vi "_script_fix_Parse State Queue in Find Parse State Queue vi name.vi"   [LabVIEW 2014]
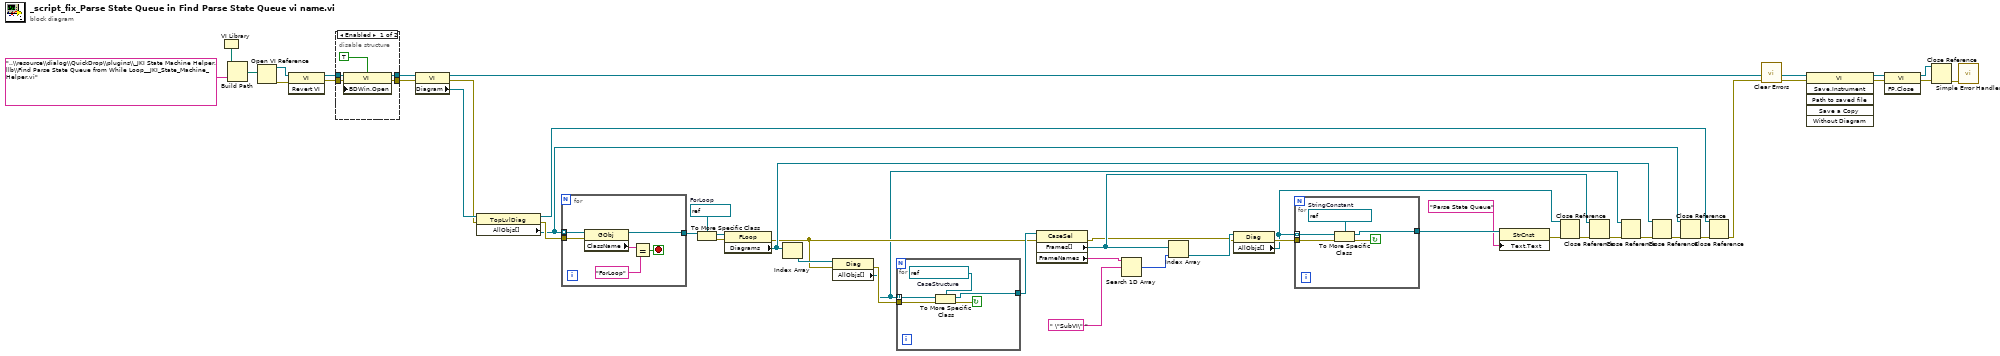
[diagram p0: block diagram]
diagram:
  w37 = refnum<vi> refnum  # ForLoop
  n1 = VI Library() -> (path=w46:path)
  n2 = Build Path(base path=w46, name or relative path="..\\resource\\dialog\\QuickDrop\\plugins\\_JKI State Machine Helper.llb\\Find Parse State Queue from While Loop__JKI_State_Machine_Helper.vi") -> (appended path=w44:path)
  n3 = Open VI Reference(vi path=w44) -> (vi reference=w47:refnum<vi>, error out=w48:errorcluster)  [unwired: 5 in]
  n4 = invoke class="VI" method="Revert VI"(reference=w47, error in=w48) -> (reference out=w24:refnum<vi>, error out=w23:errorcluster)  [unwired: 1 in, 1 out]
  n5 = disable-structure shown="Enabled" {
    disable-tunnel: w24 -> [w53 w55]
    disable-tunnel: w23 -> [w52 w54]
    disable-tunnel: [w51 w55] -> w22
    disable-tunnel: [w50 w54] -> w21
    frame Enabled {
      n6 = property class="VI"(reference=w53, error in=w52, "BDWin.Open"=TRUE ("Block Diagram Window:Open")) -> (reference out=w51:refnum<vi>, error out=w50:errorcluster)
    }
    frame Disabled {
    }
  }
  n7 = property class="VI"(reference=w22, error in=w21) -> (reference out=w43:refnum<vi>, error out=w40:errorcluster, "Diagram"=w41:refnum<vi>)
  n8 = property class="TopLvlDiag"(reference=w41, error in=w40) -> (reference out=w26:refnum<vi>, error out=w39:errorcluster, "AllObjs[]"=w28:refnum<vi>[])
  n9 = for {
    tunnel: w28 -> [w61] mode=indexing
    tunnel: w39 -> [w60]
    tunnel: [w59] -> w38
    stop <- w56 stop-if-true
    n10 = property class="GObj"(reference=w61, error in=w60) -> (reference out=w59:refnum<vi>, "ClassName"=w58:string)  [unwired: 1 out]
    n11 = Equal?(x=w58, y="ForLoop") -> (x = y?=w56:bool)
  }
  n12 = To More Specific Class(target class=w37, reference=w38) -> (specific class reference=w36:refnum<vi>, error out=w35:errorcluster)  [unwired: 1 in]
  n13 = property class="FLoop"(reference=w36, error in=w35) -> (error out=w16:errorcluster, "Diagrams"=w20:refnum<vi>[])  [unwired: 1 out]
  n14 = Index Array(array=w20) -> (element=w19:refnum<vi>)  [unwired: 1 in]
  n15 = property class="Diag"(reference=w19, error in=w16) -> (error out=w18:errorcluster, "AllObjs[]"=w12:refnum<vi>[])  [unwired: 1 out]
  n16 = for {
    tunnel: w12 -> [w66] mode=indexing
    tunnel: w18 -> [w65]
    tunnel: [w63] -> w17
    stop <- w64 continue-if-true
    w62 = refnum<vi> refnum  # CaseStructure
    n17 = To More Specific Class(target class=w62, reference=w66, error in=w65) -> (specific class reference=w63:refnum<vi>, error out=w64:errorcluster)
  }
  n18 = property class="CaseSel"(reference=w17, error in=w16) -> (error out=w6:errorcluster, "Frames[]"=w9:refnum<vi>[], "FrameNames"=w11:string[])  [unwired: 1 out]
  n19 = Search 1D Array(1D array=w11, element=" \"SubVI\" " ("y")) -> (index of element=w8:i32)  [unwired: 1 in]
  n20 = Index Array(array=w9, index=w8) -> (element=w7:refnum<vi>)
  n21 = property class="Diag"(reference=w7, error in=w6) -> (error out=w34:errorcluster, "AllObjs[]"=w30:refnum<vi>[])  [unwired: 1 out]
  n22 = for {
    tunnel: w30 -> [w71] mode=indexing
    tunnel: w34 -> [w70]
    tunnel: [w67] -> w33
    stop <- w68 continue-if-true
    w69 = refnum<vi> refnum  # StringConstant
    n23 = To More Specific Class(target class=w69, reference=w71, error in=w70) -> (specific class reference=w67:refnum<vi>, error out=w68:errorcluster)
  }
  n24 = property class="StrCnst"(reference=w33, "Text.Text"="Parse State Queue") -> (error out=w31:errorcluster)  [unwired: 1 in, 1 out]
  n25 = Close Reference(reference=w30, error in (no error)=w31) -> (error out=w15:errorcluster)
  n26 = Close Reference(reference=w9, error in (no error)=w15) -> (error out=w14:errorcluster)
  n27 = Close Reference(reference=w12, error in (no error)=w14) -> (error out=w13:errorcluster)
  n28 = Close Reference(reference=w20, error in (no error)=w13) -> (error out=w29:errorcluster)
  n29 = Close Reference(reference=w28, error in (no error)=w29) -> (error out=w27:errorcluster)
  n30 = Close Reference(reference=w26, error in (no error)=w27) -> (error out=w25:errorcluster)
  n31 = call <vilib>:"Clear Errors.vi"("error in (no error)"=w25) -> ("error out"=w1:errorcluster)  [unwired: 6 in]
  n32 = invoke class="VI" method="Save.Instrument"(reference=w43, error in=w1) -> (reference out=w3:refnum<vi>, error out=w5:errorcluster)  [unwired: 4 in, 4 out]
  n33 = invoke class="VI" method="FP.Close"(reference=w3, error in=w5) -> (reference out=w2:refnum<vi>, error out=w4:errorcluster)  [unwired: 1 in, 1 out]
  n34 = Close Reference(reference=w2, error in (no error)=w4) -> (error out=w42:errorcluster)
  n35 = call <vilib>:"Simple Error Handler.vi"("error in (no error)"=w42) -> ()  [unwired: 4 in, 5 out]
